vi "selectData.vi"(8 "error in (no error)":errorcluster, 11 "AllData":T2) -> (0 "error out":errorcluster, 3 "?":T1={"ControlFlag"=TRUE, "Fx"=0.0, "Fy"=0.0, "Theta0"=0.0, "Theta1"=0.0, "CurrentX"=0.0, "CurrentY"=0.0, "TargetX"=0.0, "TargetY"=0.0, "DeadZone"=0.0, "Assistance?"=FALSE, "AssitanceLevel"=0.0})   [LabVIEW 2017, in "admittanceControllerLibrary.lvlib"]
doc: "This VI takes in All the data and selects the necessary data for use with the low level control module."
uses:
  admittanceControllerLibrary.lvlib
  TypeDefs/allData.ctl
  TypeDefs/dataOut.ctl
  TypeDefs/dataIn.ctl
  Controls/ControlVariables.ctl
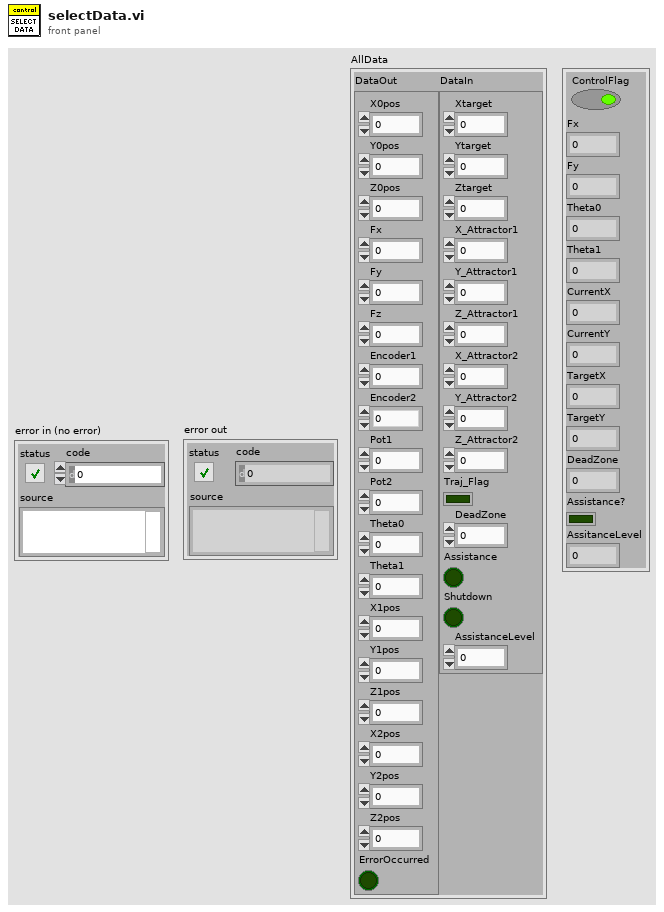
[diagram p1: front panel]
types:
  T1 = typedef "admittanceControllerLibrary.lvlib/ControlVariables.ctl" = cluster{"ControlFlag":bool, "Fx":dbl, "Fy":dbl, "Theta0":dbl, "Theta1":dbl, "CurrentX":dbl, "CurrentY":dbl, "TargetX":dbl, "TargetY":dbl, "DeadZone":dbl, "Assistance?":bool, "AssitanceLevel":dbl}
  T2 = typedef "allData.ctl" = cluster{"DataOut":T3, "DataIn":T4}
  T3 = typedef "dataOut.ctl" = cluster{"X0pos":dbl, "Y0pos":dbl, "Z0pos":dbl, "Fx":dbl, "Fy":dbl, "Fz":dbl, "Encoder1":i32, "Encoder2":i32, "Pot1":dbl, "Pot2":dbl, "Theta0":dbl, "Theta1":dbl, "X1pos":dbl, "Y1pos":dbl, "Z1pos":dbl, "X2pos":dbl, "Y2pos":dbl, "Z2pos":dbl, "ErrorOccurred":bool}
  T4 = typedef "dataIn.ctl" = cluster{"Xtarget":dbl, "Ytarget":dbl, "Ztarget":dbl, "X_Attractor1":dbl, "Y_Attractor1":dbl, "Z_Attractor1":dbl, "X_Attractor2":dbl, "Y_Attractor2":dbl, "Z_Attractor2":dbl, "Traj_Flag":bool, "DeadZone":dbl, "Assistance":bool, "Shutdown":bool, "AssistanceLevel":dbl}
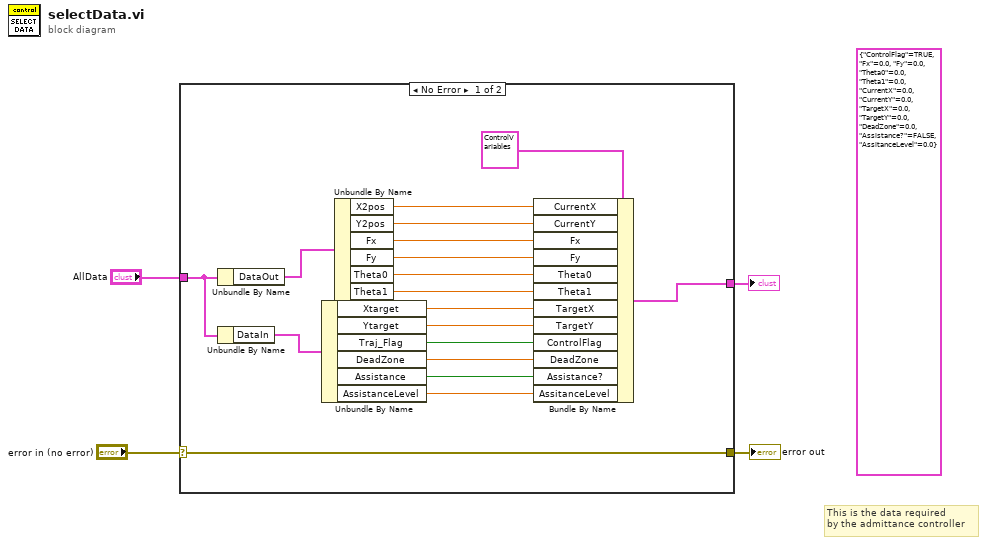
[diagram p0: block diagram]
diagram:
  (unwired) T1 {"ControlFlag"=TRUE, "Fx"=0.0, "Fy"=0.0, "Theta0"=0.0, "Theta1"=0.0, "CurrentX"=0.0, "CurrentY"=0.0, "TargetX"=0.0, "TargetY"=0.0, "DeadZone"=0.0, "Assistance?"=FALSE, "AssitanceLevel"=0.0}
  # "This is the data required\nby the admittance controller"
  n1 = case shown="No Error" "error in (no error)" {
    selector: "error in (no error)" -> [w20 w23]
    tunnel: [w20 w23] -> w3
    tunnel: "AllData" -> [w14 _]
    tunnel: [w21 _] -> w1
    frame No Error {
      n2 = Unbundle By Name(w14) -> ("DataOut"=w19:T3)
      n3 = Unbundle By Name(w14) -> ("DataIn"=w13:T4)
      n4 = Unbundle By Name(w13) -> ("Xtarget"=w10:dbl, "Ytarget"=w9:dbl, "Traj_Flag"=w8:bool, "DeadZone"=w7:dbl, "Assistance"=w6:bool, "AssistanceLevel"=w5:dbl)
      n5 = Unbundle By Name(w19) -> ("X2pos"=w18:dbl, "Y2pos"=w17:dbl, "Fx"=w16:dbl, "Fy"=w15:dbl, "Theta0"=w12:dbl, "Theta1"=w11:dbl)
      n6 = Bundle By Name(cluster=T1 {"ControlFlag"=TRUE, "Fx"=0.0, "Fy"=0.0, "Theta0"=0.0, "Theta1"=0.0, "CurrentX"=0.0, "CurrentY"=0.0, "TargetX"=0.0, "TargetY"=0.0, "DeadZone"=0.0, "Assistance?"=FALSE, "AssitanceLevel"=0.0}, "CurrentX"=w18, "CurrentY"=w17, "Fx"=w16, "Fy"=w15, "Theta0"=w12, "Theta1"=w11, "TargetX"=w10, "TargetY"=w9, "ControlFlag"=w8, "DeadZone"=w7, "Assistance?"=w6, "AssitanceLevel"=w5) -> (w21:T1)
    }
    frame Error {
    }
  }
  "error out" <- w3
  "?" <- w1
